vi "GetCAENState.vi"(10 "error in (no error)":errorcluster, 11 "TCP Session":refnum<k5>) -> (0 "error out":errorcluster, 1 "Switch Heater":bool, 2 "Enum":T1(ring), 3 "TCP Session Out":refnum<k5>)   [LabVIEW 2025]
doc: "Author: Scott Hannahs <sth@magnet.fsu.edu>\n\nThis software is licensed for use under the “MIT License\"\nCopyright (c) 2025 Scott Hannahs, sth@sth@magnet.sthnet.net\n\nPermission is hereby granted, free of charge, to any person obtaining a copy of this software and associated documentation files (the \"Software\"), to deal in the Software without restriction, including without limitation the rights to use, copy, modify, merge, publish, distribute, sublicense, and/or sell copies of the Software, and to permit persons to whom the Software is furnished to do so, subject to the following conditions: The above copyright notice and this permission notice shall be included in all copies or substantial portions of the Software.\n\nTHE SOFTWARE IS PROVIDED \"AS IS\", WITHOUT WARRANTY OF ANY KIND, EXPRESS OR IMPLIED, INCLUDING BUT NOT LIMITED TO THE WARRANTIES OF MERCHANTABILITY, FITNESS FOR A PARTICULAR PURPOSE AND NONINFRINGEMENT. IN NO EVENT SHALL THE AUTHORS OR COPYRIGHT HOLDERS BE LIABLE FOR ANY CLAIM, DAMAGES OR OTHER LIABILITY, WHETHER IN AN ACTION OF CONTRACT, TORT OR OTHERWISE, ARISING FROM, OUT OF OR IN CONNECTION WITH THE SOFTWARE OR THE USE OR OTHER DEALINGS IN THE SOFTWARE."
panel:
  out "Binary Status Array":bool[](array[boolean])
  out "Raw Status String":string
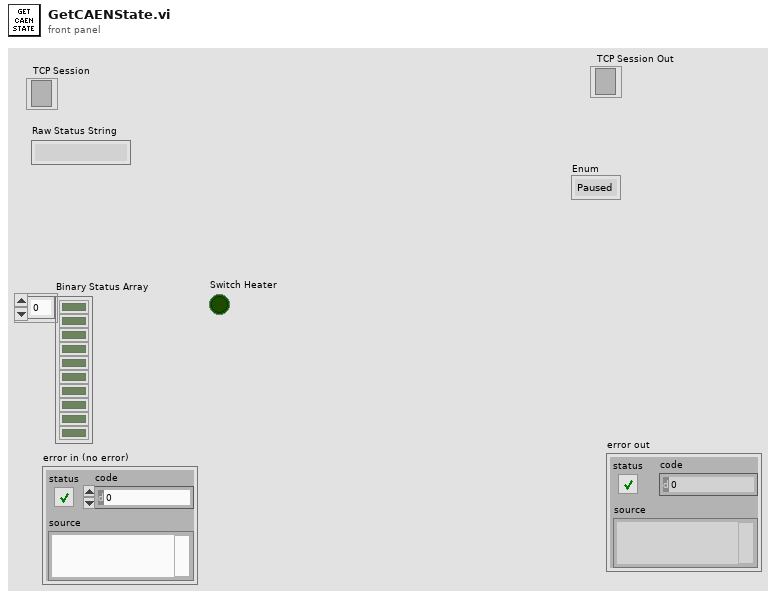
[diagram p1: front panel]
types:
  T1 = enum16{"Paused", "Ramping to Programmed Field", "QUENCH"}
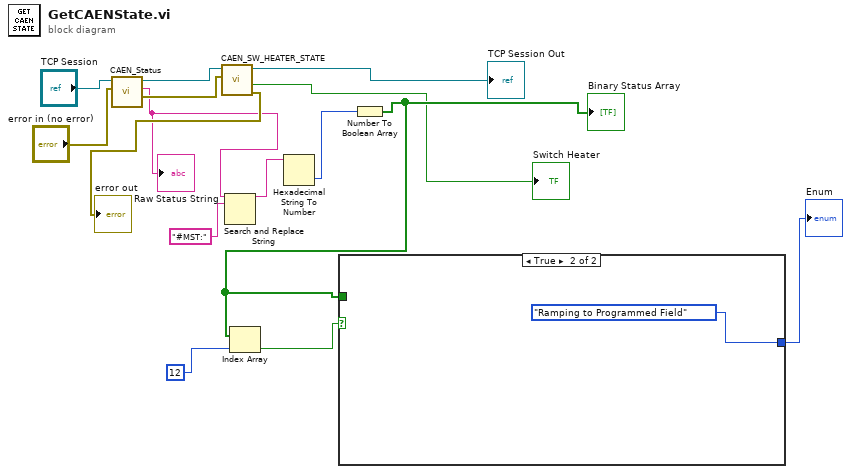
[diagram p0: block diagram]
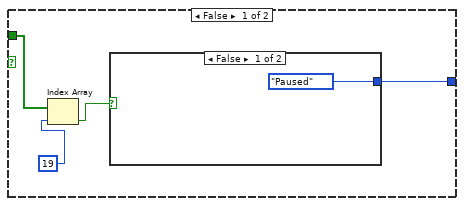
[diagram p2: hidden frame]
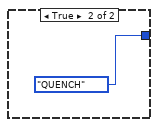
[diagram p3: hidden frame]
diagram:
  n1 = call "CAEN_Status.vi"("error in (no error)"="error in (no error)", "TCP Network Connection Refnum"="TCP Session") -> ("error out"=w7:errorcluster, "String"=w2:string, "TCP Network Connection Refnum 2"=w8:refnum<k5>)  [unwired: 7 in]
  "Raw Status String" <- w2
  n2 = call "CAEN_SW_HEATER_STATE.vi"("error in (no error)"=w7, "Network Session"=w8) -> ("error out"=→"error out":errorcluster, "SW Heater"=→"Switch Heater":bool, "Network Session Out"=→"TCP Session Out":refnum<k5>)  [unwired: 6 in, 1 out]
  n3 = Search and Replace String(input string=w2, search string="#MST:") -> (result string=w1:string)  [unwired: 6 in, 3 out]
  n4 = Hexadecimal String To Number(string=w1) -> (number=w15:u32)  [unwired: 2 in, 1 out]
  n5 = Number To Boolean Array(number=w15) -> (Boolean array=w10:bool[])
  "Binary Status Array" <- w10
  n6 = Index Array(array=w10, index=12) -> (element=w11:bool)
  n7 = case shown="True" w11 {
    tunnel: w10 -> [w19 _]
    tunnel: [w16 T1."Ramping to Programmed Field" ("Enum")] -> w9
    frame False {
      n8 = Index Array(array=w19, index=19) -> (element=w17:bool)
      n9 = case shown="False" w17 {
        tunnel: [T1."Paused" ("Enum") T1."QUENCH" ("Enum")] -> w16
        frame False {
        }
        frame True {
        }
      }
    }
    frame True {
    }
  }
  "Enum" <- w9
